vi "Read don't grow FP.vi"(8 "error in (no error)":errorcluster, 11 "cosmetic changes in":refnum<class "cosmetic changes.lvclass">) -> (0 "error out":errorcluster, 2 "don't grow FP":bool, 3 "cosmetic changes out":refnum<class "cosmetic changes.lvclass">)   [LabVIEW 2013, in "cosmetic changes.lvclass"]
uses:
  cosmetic changes.lvclass
  cosmetic changes.lvclass/cosmetic changes.ctl
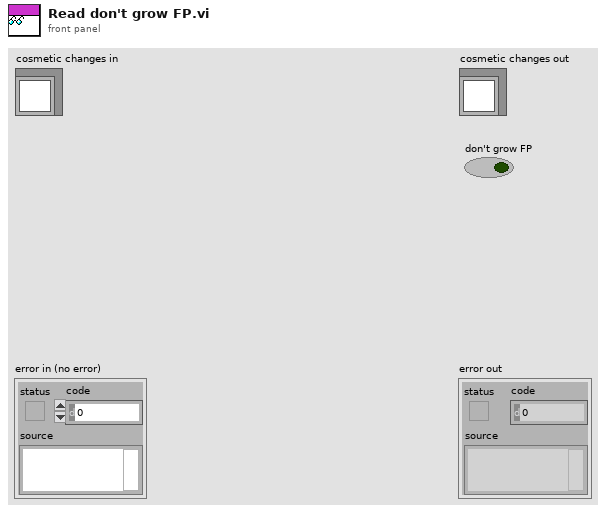
[diagram p1: front panel]
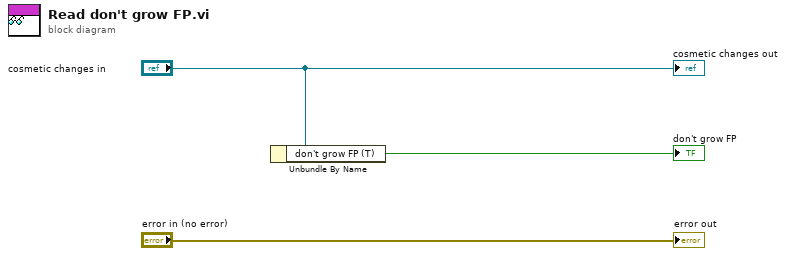
[diagram p0: block diagram]
diagram:
  n1 = Unbundle By Name("cosmetic changes in") -> ("don't grow FP (T)"=→"don't grow FP":bool)
  "error out" <- "error in (no error)"
  "cosmetic changes out" <- "cosmetic changes in"
